vi "Write Text.vi"(8 "error in (no error)":errorcluster, 9 "String":string, 10 "timeout ms (5000)":i32=5000, 11 "Websocket Handler in":refnum<class "Websocket Handler.lvclass">) -> (0 "error out":errorcluster, 3 "Websocket Handler out":refnum<class "Websocket Handler.lvclass">)   [LabVIEW 2020, in "wamplv.lvlib" / "Websocket Handler.lvclass"]
uses:
  Websocket Handler.lvclass
  Websocket Handler.lvclass/Websocket Handler.ctl
  <vilib>/MediaMongrels Ltd/WebSockets/WebSockets/WebSocket Client/WebSocket Client.lvclass
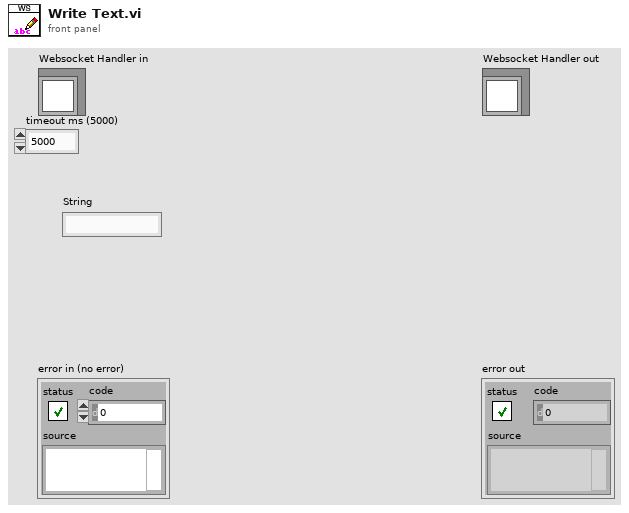
[diagram p1: front panel]
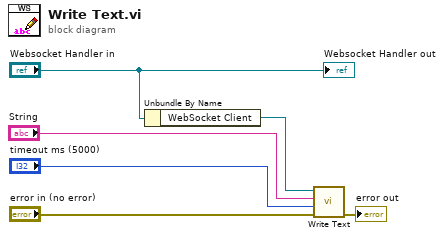
[diagram p0: block diagram]
diagram:
  n1 = Unbundle By Name("Websocket Handler in") -> ("WebSocket Client"=w3:refnum<class "WebSocket Client.lvclass">)
  n2 = call-dynamic "Write Text.vi"("error in (no error)"="error in (no error)", "timeout ms (5000)"="timeout ms (5000)", "String Data"="String", "WebSocket in"=w3) -> ("error out"=→"error out":errorcluster)  [unwired: 6 in, 1 out]
  "Websocket Handler out" <- "Websocket Handler in"
